vi "Topmost VI Reference.vi"() -> (1 "Topmost VI's Reference":refnum<vi>)   [LabVIEW 2017]
doc: "Returns a reference to the top-level VI in the current call chain."
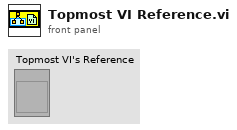
[diagram p1: front panel]
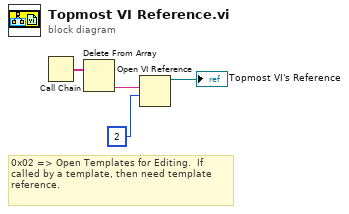
[diagram p0: block diagram]
diagram:
  # "0x02 => Open Templates for Editing.  If called by a template, then need template reference."
  n1 = Call Chain() -> (call chain=w4:string[])
  n2 = Delete From Array(array=w4) -> (deleted portion=w3:string)  [unwired: 2 in, 1 out]
  n3 = Open VI Reference(vi path=w3, options=2) -> (vi reference=→"Topmost VI's Reference":refnum<vi>)  [unwired: 4 in, 1 out]
